vi "addDestination.vi"(8 "Error In":errorcluster, 10 "filePath":string, 11 "QWinJumpListCategory In":refnum<class "QWinJumpListCategory.lvclass">) -> (0 "Error Out":errorcluster, 2 "Value":refnum<class "QWinJumpListItem.lvclass">, 3 "QWinJumpListCategory Out":refnum<class "QWinJumpListCategory.lvclass">)   [LabVIEW 2014, in "QWinJumpListCategory.lvclass"]
doc: "LabVIEW-specific documentation is not yet available. See <b>https://doc.qt.io/qt-5/qwinjumplistcategory.html#addDestination</b>"
uses:
  QWinJumpListCategory.lvclass
  QWinJumpListItem/QWinJumpListItem.lvclass
  LQ Core/LQIdentity/LQIdentity.lvclass/LQIdentity.ctl
  LQ Core/LQ Core.lvlib
  LQ Core/LQIdentity/LQIdentity.lvclass
  LQ Core/LQCoreEngine/LQCoreEngine.lvclass
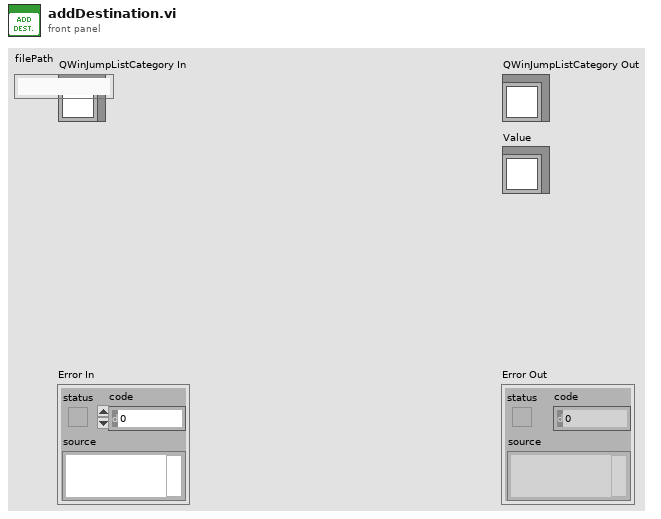
[diagram p1: front panel]
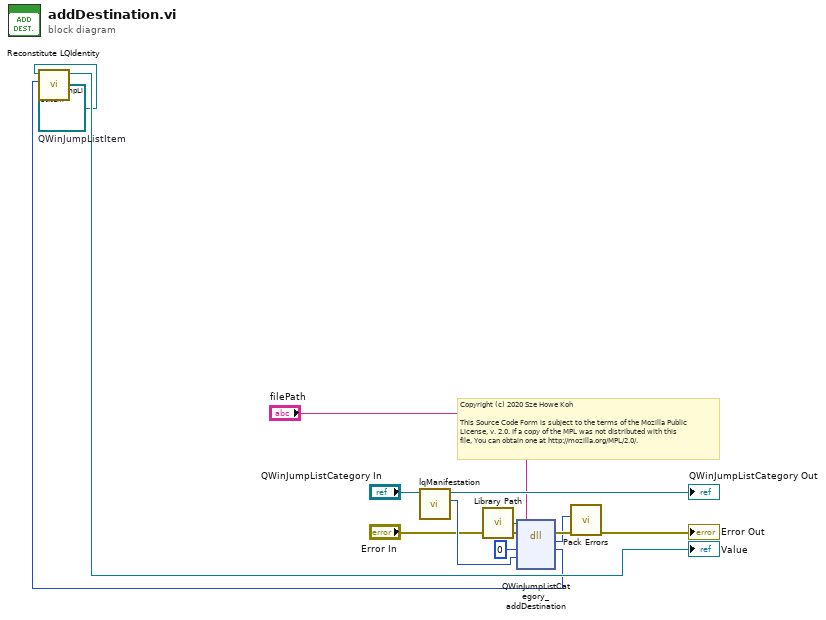
[diagram p0: block diagram]
diagram:
  w2 = refnum<class "QWinJumpListItem.lvclass"> refnum  # QWinJumpListItem
  # "Copyright (c) 2020 Sze Howe Koh\n\nThis Source Code Form is subject to the terms of the Mozilla Public\nLicense, v. 2.0. If a copy of the MPL was not distributed with this\nfile, You can obtain one at http://mozilla.org/MPL/2.0/."
  n1 = call "lqManifestation.vi"("LQIdentity in"="QWinJumpListCategory In") -> ("Manifestation"=w9:u64, "LQIdentity out"=→"QWinJumpListCategory Out":refnum<class "QWinJumpListCategory.lvclass">)  [unwired: 9 in]
  n2 = call "Library Path.vi"() -> ("Library Path"=w10:path)
  n3 = dll-call lib="?" fn="QWinJumpListCategory_addDestination"(path in=w10, error in="Error In", "_retVal"=u64 0 ("retVal"), "_instance"=w9, "filePath"="filePath") -> (error out=w7:errorcluster, w5:i32, "_retVal"=w3:u64)  [unwired: 3 in, 1 out]
  n4 = call "Reconstitute LQIdentity.vi"("Manifestation"=w3, "LQIdentity Prototype"=w2) -> ("Reconstituted LQIdentity"=→"Value":refnum<class "QWinJumpListItem.lvclass">)  [unwired: 8 in, 1 out]
  n5 = call "Pack Errors.vi"("Error In"=w7, "Error Code"=w5) -> ("Error Out"=→"Error Out":errorcluster)  [unwired: 9 in]
